vi "ZlutaVanoceVanoce.vi"(11 "NXT/EV3":T1) -> (3 "NXT/EV3 2":T1)   [LabVIEW 2016]
uses:
  <vilib>/NXT/Subs/LVHSConnector.ctl
  <vilib>/NXT/LegoClasses/BrickReference/BrickReference.lvclass
  <vilib>/NXT/Dual Mode Library/Display/drawText_Center.vi
  <vilib>/NXT/Dual Mode Library/Sound/PlayC.vi
  <vilib>/NXT/Dual Mode Library/Sound/PlayA.vi
  <vilib>/NXT/Dual Mode Library/Sound/PlayG.vi
  <vilib>/NXT/Dual Mode Library/Sound/PlayE.vi
  <vilib>/NXT/Dual Mode Library/Sound/PlayD.vi
  <vilib>/NXT/Dual Mode Library/Waits/Wait_Num.vi
  <vilib>/NXT/Dual Mode Library/Sound/PlayB.vi
  <vilib>/NXT/Dual Mode Library/Sound/PlayF.vi
  <vilib>/NXT/Dual Mode Library/Sound/PlayFsharp.vi
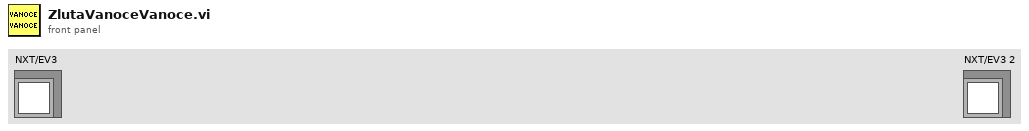
[diagram p1: front panel]
types:
  T1 = typedef "LVHSConnector.ctl" = refnum<class "BrickReference.lvclass">
diagram:
  w7 = u16 5 items=["3"=3, "4"=4, "5"=5, "6"=6, "7"=7] ("Octave")
  w8 = u16 4 items=["3"=3, "4"=4, "5"=5, "6"=6, "7"=7] ("Octave")
  w9 = u16 4 items=["3"=3, "4"=4, "5"=5, "6"=6, "7"=7] ("Octave")
  w10 = u16 4 items=["3"=3, "4"=4, "5"=5, "6"=6, "7"=7] ("Octave")
  w20 = u16 4 items=["3"=3, "4"=4, "5"=5, "6"=6, "7"=7] ("Octave")
  w19 = u16 4 items=["3"=3, "4"=4, "5"=5, "6"=6, "7"=7] ("Octave")
  w47 = u16 4 items=["3"=3, "4"=4, "5"=5, "6"=6, "7"=7] ("Octave")
  w45 = u16 4 items=["3"=3, "4"=4, "5"=5, "6"=6, "7"=7] ("Octave")
  w40 = u16 4 items=["3"=3, "4"=4, "5"=5, "6"=6, "7"=7] ("Octave")
  w39 = u16 4 items=["3"=3, "4"=4, "5"=5, "6"=6, "7"=7] ("Octave")
  w34 = u16 4 items=["3"=3, "4"=4, "5"=5, "6"=6, "7"=7] ("Octave")
  w33 = u16 4 items=["3"=3, "4"=4, "5"=5, "6"=6, "7"=7] ("Octave")
  w32 = u16 4 items=["3"=3, "4"=4, "5"=5, "6"=6, "7"=7] ("Octave")
  w27 = u16 4 items=["3"=3, "4"=4, "5"=5, "6"=6, "7"=7] ("Octave")
  w24 = u16 5 items=["3"=3, "4"=4, "5"=5, "6"=6, "7"=7] ("Octave")
  w23 = u16 5 items=["3"=3, "4"=4, "5"=5, "6"=6, "7"=7] ("Octave")
  w52 = u16 4 items=["3"=3, "4"=4, "5"=5, "6"=6, "7"=7] ("Octave")
  w53 = u16 4 items=["3"=3, "4"=4, "5"=5, "6"=6, "7"=7] ("Octave")
  w54 = u16 4 items=["3"=3, "4"=4, "5"=5, "6"=6, "7"=7] ("Octave")
  w68 = u16 4 items=["3"=3, "4"=4, "5"=5, "6"=6, "7"=7] ("Octave")
  w69 = u16 4 items=["3"=3, "4"=4, "5"=5, "6"=6, "7"=7] ("Octave")
  w70 = u16 4 items=["3"=3, "4"=4, "5"=5, "6"=6, "7"=7] ("Octave")
  w71 = u16 4 items=["3"=3, "4"=4, "5"=5, "6"=6, "7"=7] ("Octave")
  w72 = u16 4 items=["3"=3, "4"=4, "5"=5, "6"=6, "7"=7] ("Octave")
  w73 = u16 4 items=["3"=3, "4"=4, "5"=5, "6"=6, "7"=7] ("Octave")
  w85 = u16 4 items=["3"=3, "4"=4, "5"=5, "6"=6, "7"=7] ("Octave")
  w87 = u16 4 items=["3"=3, "4"=4, "5"=5, "6"=6, "7"=7] ("Octave")
  w92 = u16 4 items=["3"=3, "4"=4, "5"=5, "6"=6, "7"=7] ("Octave")
  w93 = u16 4 items=["3"=3, "4"=4, "5"=5, "6"=6, "7"=7] ("Octave")
  w98 = u16 4 items=["3"=3, "4"=4, "5"=5, "6"=6, "7"=7] ("Octave")
  w99 = u16 4 items=["3"=3, "4"=4, "5"=5, "6"=6, "7"=7] ("Octave")
  w100 = u16 4 items=["3"=3, "4"=4, "5"=5, "6"=6, "7"=7] ("Octave")
  w106 = u16 4 items=["3"=3, "4"=4, "5"=5, "6"=6, "7"=7] ("Octave")
  w109 = u16 5 items=["3"=3, "4"=4, "5"=5, "6"=6, "7"=7] ("Octave")
  w110 = u16 5 items=["3"=3, "4"=4, "5"=5, "6"=6, "7"=7] ("Octave")
  w115 = u16 4 items=["3"=3, "4"=4, "5"=5, "6"=6, "7"=7] ("Octave")
  w118 = u16 4 items=["3"=3, "4"=4, "5"=5, "6"=6, "7"=7] ("Octave")
  w119 = u16 4 items=["3"=3, "4"=4, "5"=5, "6"=6, "7"=7] ("Octave")
  w145 = u16 4 items=["3"=3, "4"=4, "5"=5, "6"=6, "7"=7] ("Octave")
  w149 = u16 4 items=["3"=3, "4"=4, "5"=5, "6"=6, "7"=7] ("Octave")
  w146 = u16 4 items=["3"=3, "4"=4, "5"=5, "6"=6, "7"=7] ("Octave")
  w138 = u16 4 items=["3"=3, "4"=4, "5"=5, "6"=6, "7"=7] ("Octave")
  w135 = u16 4 items=["3"=3, "4"=4, "5"=5, "6"=6, "7"=7] ("Octave")
  w130 = u16 4 items=["3"=3, "4"=4, "5"=5, "6"=6, "7"=7] ("Octave")
  w133 = u16 4 items=["3"=3, "4"=4, "5"=5, "6"=6, "7"=7] ("Octave")
  w125 = u16 4 items=["3"=3, "4"=4, "5"=5, "6"=6, "7"=7] ("Octave")
  w122 = u16 4 items=["3"=3, "4"=4, "5"=5, "6"=6, "7"=7] ("Octave")
  w121 = u16 4 items=["3"=3, "4"=4, "5"=5, "6"=6, "7"=7] ("Octave")
  w167 = u16 4 items=["3"=3, "4"=4, "5"=5, "6"=6, "7"=7] ("Octave")
  w164 = u16 4 items=["3"=3, "4"=4, "5"=5, "6"=6, "7"=7] ("Octave")
  w160 = u16 4 items=["3"=3, "4"=4, "5"=5, "6"=6, "7"=7] ("Octave")
  w163 = u16 4 items=["3"=3, "4"=4, "5"=5, "6"=6, "7"=7] ("Octave")
  w175 = u16 4 items=["3"=3, "4"=4, "5"=5, "6"=6, "7"=7] ("Octave")
  w178 = u16 4 items=["3"=3, "4"=4, "5"=5, "6"=6, "7"=7] ("Octave")
  w183 = u16 4 items=["3"=3, "4"=4, "5"=5, "6"=6, "7"=7] ("Octave")
  w180 = u16 4 items=["3"=3, "4"=4, "5"=5, "6"=6, "7"=7] ("Octave")
  w188 = u16 4 items=["3"=3, "4"=4, "5"=5, "6"=6, "7"=7] ("Octave")
  w191 = u16 4 items=["3"=3, "4"=4, "5"=5, "6"=6, "7"=7] ("Octave")
  w192 = u16 4 items=["3"=3, "4"=4, "5"=5, "6"=6, "7"=7] ("Octave")
  w195 = u16 4 items=["3"=3, "4"=4, "5"=5, "6"=6, "7"=7] ("Octave")
  w203 = u16 5 items=["3"=3, "4"=4, "5"=5, "6"=6, "7"=7] ("Octave")
  w204 = u16 4 items=["3"=3, "4"=4, "5"=5, "6"=6, "7"=7] ("Octave")
  w205 = u16 4 items=["3"=3, "4"=4, "5"=5, "6"=6, "7"=7] ("Octave")
  w206 = u16 4 items=["3"=3, "4"=4, "5"=5, "6"=6, "7"=7] ("Octave")
  w216 = u16 4 items=["3"=3, "4"=4, "5"=5, "6"=6, "7"=7] ("Octave")
  w215 = u16 4 items=["3"=3, "4"=4, "5"=5, "6"=6, "7"=7] ("Octave")
  w243 = u16 4 items=["3"=3, "4"=4, "5"=5, "6"=6, "7"=7] ("Octave")
  w241 = u16 4 items=["3"=3, "4"=4, "5"=5, "6"=6, "7"=7] ("Octave")
  w236 = u16 4 items=["3"=3, "4"=4, "5"=5, "6"=6, "7"=7] ("Octave")
  w235 = u16 4 items=["3"=3, "4"=4, "5"=5, "6"=6, "7"=7] ("Octave")
  w230 = u16 4 items=["3"=3, "4"=4, "5"=5, "6"=6, "7"=7] ("Octave")
  w229 = u16 4 items=["3"=3, "4"=4, "5"=5, "6"=6, "7"=7] ("Octave")
  w228 = u16 4 items=["3"=3, "4"=4, "5"=5, "6"=6, "7"=7] ("Octave")
  w223 = u16 4 items=["3"=3, "4"=4, "5"=5, "6"=6, "7"=7] ("Octave")
  w220 = u16 5 items=["3"=3, "4"=4, "5"=5, "6"=6, "7"=7] ("Octave")
  w219 = u16 5 items=["3"=3, "4"=4, "5"=5, "6"=6, "7"=7] ("Octave")
  w248 = u16 4 items=["3"=3, "4"=4, "5"=5, "6"=6, "7"=7] ("Octave")
  w249 = u16 4 items=["3"=3, "4"=4, "5"=5, "6"=6, "7"=7] ("Octave")
  w250 = u16 4 items=["3"=3, "4"=4, "5"=5, "6"=6, "7"=7] ("Octave")
  w264 = u16 4 items=["3"=3, "4"=4, "5"=5, "6"=6, "7"=7] ("Octave")
  w265 = u16 4 items=["3"=3, "4"=4, "5"=5, "6"=6, "7"=7] ("Octave")
  w266 = u16 4 items=["3"=3, "4"=4, "5"=5, "6"=6, "7"=7] ("Octave")
  w267 = u16 4 items=["3"=3, "4"=4, "5"=5, "6"=6, "7"=7] ("Octave")
  w268 = u16 4 items=["3"=3, "4"=4, "5"=5, "6"=6, "7"=7] ("Octave")
  w269 = u16 4 items=["3"=3, "4"=4, "5"=5, "6"=6, "7"=7] ("Octave")
  w279 = i16 0 items=["1", "2", "3", "4", "5", "6", "7", "8", "9", "10", "11", "12"] ("Line")
  w283 = u16 4 items=["3"=3, "4"=4, "5"=5, "6"=6, "7"=7] ("Octave")
  w285 = u16 4 items=["3"=3, "4"=4, "5"=5, "6"=6, "7"=7] ("Octave")
  w290 = u16 4 items=["3"=3, "4"=4, "5"=5, "6"=6, "7"=7] ("Octave")
  w291 = u16 4 items=["3"=3, "4"=4, "5"=5, "6"=6, "7"=7] ("Octave")
  w296 = u16 4 items=["3"=3, "4"=4, "5"=5, "6"=6, "7"=7] ("Octave")
  w297 = u16 4 items=["3"=3, "4"=4, "5"=5, "6"=6, "7"=7] ("Octave")
  w298 = u16 4 items=["3"=3, "4"=4, "5"=5, "6"=6, "7"=7] ("Octave")
  w304 = u16 4 items=["3"=3, "4"=4, "5"=5, "6"=6, "7"=7] ("Octave")
  w307 = u16 5 items=["3"=3, "4"=4, "5"=5, "6"=6, "7"=7] ("Octave")
  w308 = u16 5 items=["3"=3, "4"=4, "5"=5, "6"=6, "7"=7] ("Octave")
  n1 = call-poly <vilib>:"PolyDisplay.vi"("Text"="\n\n\n\n\nEV3 JUK3BOX:\nVanoce, Vanoce\n\n\n\n\n\n", "NXT/EV3"="NXT/EV3", "Line"=w279) -> ("NXT/EV3"=w196:T1)  [unwired: 1 in]
  n2 = call-poly <vilib>:"PolySound.vi"("Duration (500 ms)"=u16 1000, "NXT/EV3"=w196, "Octave"=w308) -> ("NXT/EV3"=w303:T1)  [unwired: 1 in]
  n3 = call-poly <vilib>:"PolySound.vi"("Duration (500 ms)"=u16 500, "NXT/EV3"=w303, "Octave"=w307) -> ("NXT/EV3"=w302:T1)  [unwired: 1 in]
  n4 = call-poly <vilib>:"PolySound.vi"("Duration (500 ms)"=u16 500, "NXT/EV3"=w302, "Octave"=w304) -> ("NXT/EV3"=w301:T1)  [unwired: 1 in]
  n5 = call-poly <vilib>:"PolySound.vi"("Duration (500 ms)"=u16 1000, "NXT/EV3"=w301, "Octave"=w298) -> ("NXT/EV3"=w300:T1)  [unwired: 1 in]
  n6 = call-poly <vilib>:"PolySound.vi"("Duration (500 ms)"=u16 500, "NXT/EV3"=w300, "Octave"=w297) -> ("NXT/EV3"=w299:T1)  [unwired: 1 in]
  n7 = call-poly <vilib>:"PolySound.vi"("Duration (500 ms)"=u16 500, "NXT/EV3"=w299, "Octave"=w296) -> ("NXT/EV3"=w288:T1)  [unwired: 1 in]
  n8 = call-poly <vilib>:"PolySound.vi"("Duration (500 ms)"=u16 500, "NXT/EV3"=w288, "Octave"=w291) -> ("NXT/EV3"=w287:T1)  [unwired: 1 in]
  n9 = call-poly <vilib>:"PolySound.vi"("Duration (500 ms)"=u16 1000, "NXT/EV3"=w287, "Octave"=w290) -> ("NXT/EV3"=w284:T1)  [unwired: 1 in]
  n10 = call-poly <vilib>:"PolySound.vi"("Duration (500 ms)"=u16 500, "NXT/EV3"=w284, "Octave"=w285) -> ("NXT/EV3"=w282:T1)  [unwired: 1 in]
  n11 = call-poly <vilib>:"PolySound.vi"("Duration (500 ms)"=u16 1000, "NXT/EV3"=w282, "Octave"=w283) -> ("NXT/EV3"=w261:T1)  [unwired: 1 in]
  n12 = call-poly <vilib>:"PolyWait.vi"("Time (1 sec)"=sgl 0.7, "NXT/EV3"=w261) -> ("NXT/EV3"=w260:T1)  [unwired: 2 in]
  n13 = call-poly <vilib>:"PolySound.vi"("Duration (500 ms)"=u16 500, "NXT/EV3"=w260, "Octave"=w269) -> ("NXT/EV3"=w278:T1)  [unwired: 1 in]
  n14 = call-poly <vilib>:"PolySound.vi"("Duration (500 ms)"=u16 1000, "NXT/EV3"=w278, "Octave"=w268) -> ("NXT/EV3"=w277:T1)  [unwired: 1 in]
  n15 = call-poly <vilib>:"PolySound.vi"("Duration (500 ms)"=u16 500, "NXT/EV3"=w277, "Octave"=w267) -> ("NXT/EV3"=w276:T1)  [unwired: 1 in]
  n16 = call-poly <vilib>:"PolySound.vi"("Duration (500 ms)"=u16 1000, "NXT/EV3"=w276, "Octave"=w266) -> ("NXT/EV3"=w275:T1)  [unwired: 1 in]
  n17 = call-poly <vilib>:"PolySound.vi"("Duration (500 ms)"=u16 1000, "NXT/EV3"=w275, "Octave"=w265) -> ("NXT/EV3"=w262:T1)  [unwired: 1 in]
  n18 = call-poly <vilib>:"PolySound.vi"("Duration (500 ms)"=u16 1900, "NXT/EV3"=w262, "Octave"=w264) -> ("NXT/EV3"=w258:T1)  [unwired: 1 in]
  n19 = call-poly <vilib>:"PolyWait.vi"("Time (1 sec)"=sgl 0.3, "NXT/EV3"=w258) -> ("NXT/EV3"=w256:T1)  [unwired: 2 in]
  n20 = call-poly <vilib>:"PolySound.vi"("Duration (500 ms)"=u16 500, "NXT/EV3"=w256, "Octave"=w250) -> ("NXT/EV3"=w255:T1)  [unwired: 1 in]
  n21 = call-poly <vilib>:"PolySound.vi"("Duration (500 ms)"=u16 500, "NXT/EV3"=w255, "Octave"=w249) -> ("NXT/EV3"=w254:T1)  [unwired: 1 in]
  n22 = call-poly <vilib>:"PolySound.vi"("Duration (500 ms)"=u16 500, "NXT/EV3"=w254, "Octave"=w248) -> ("NXT/EV3"=w217:T1)  [unwired: 1 in]
  n23 = call-poly <vilib>:"PolySound.vi"("Duration (500 ms)"=u16 1000, "NXT/EV3"=w217, "Octave"=w219) -> ("NXT/EV3"=w224:T1)  [unwired: 1 in]
  n24 = call-poly <vilib>:"PolySound.vi"("Duration (500 ms)"=u16 500, "NXT/EV3"=w224, "Octave"=w220) -> ("NXT/EV3"=w197:T1)  [unwired: 1 in]
  "NXT/EV3 2" <- w197
  n25 = call-poly <vilib>:"PolySound.vi"("Duration (500 ms)"=u16 500, "NXT/EV3"=w197, "Octave"=w223) -> ("NXT/EV3"=w225:T1)  [unwired: 1 in]
  n26 = call-poly <vilib>:"PolySound.vi"("Duration (500 ms)"=u16 1000, "NXT/EV3"=w225, "Octave"=w228) -> ("NXT/EV3"=w226:T1)  [unwired: 1 in]
  n27 = call-poly <vilib>:"PolySound.vi"("Duration (500 ms)"=u16 500, "NXT/EV3"=w226, "Octave"=w229) -> ("NXT/EV3"=w227:T1)  [unwired: 1 in]
  n28 = call-poly <vilib>:"PolySound.vi"("Duration (500 ms)"=u16 500, "NXT/EV3"=w227, "Octave"=w230) -> ("NXT/EV3"=w238:T1)  [unwired: 1 in]
  n29 = call-poly <vilib>:"PolySound.vi"("Duration (500 ms)"=u16 500, "NXT/EV3"=w238, "Octave"=w235) -> ("NXT/EV3"=w239:T1)  [unwired: 1 in]
  n30 = call-poly <vilib>:"PolySound.vi"("Duration (500 ms)"=u16 1000, "NXT/EV3"=w239, "Octave"=w236) -> ("NXT/EV3"=w242:T1)  [unwired: 1 in]
  n31 = call-poly <vilib>:"PolySound.vi"("Duration (500 ms)"=u16 500, "NXT/EV3"=w242, "Octave"=w241) -> ("NXT/EV3"=w244:T1)  [unwired: 1 in]
  n32 = call-poly <vilib>:"PolySound.vi"("Duration (500 ms)"=u16 1000, "NXT/EV3"=w244, "Octave"=w243) -> ("NXT/EV3"=w246:T1)  [unwired: 1 in]
  n33 = call-poly <vilib>:"PolyWait.vi"("Time (1 sec)"=sgl 0.7, "NXT/EV3"=w246) -> ("NXT/EV3"=w211:T1)  [unwired: 2 in]
  n34 = call-poly <vilib>:"PolySound.vi"("Duration (500 ms)"=u16 500, "NXT/EV3"=w211, "Octave"=w215) -> ("NXT/EV3"=w212:T1)  [unwired: 1 in]
  n35 = call-poly <vilib>:"PolySound.vi"("Duration (500 ms)"=u16 1000, "NXT/EV3"=w212, "Octave"=w216) -> ("NXT/EV3"=w210:T1)  [unwired: 1 in]
  n36 = call-poly <vilib>:"PolySound.vi"("Duration (500 ms)"=u16 500, "NXT/EV3"=w210, "Octave"=w206) -> ("NXT/EV3"=w209:T1)  [unwired: 1 in]
  n37 = call-poly <vilib>:"PolySound.vi"("Duration (500 ms)"=u16 1000, "NXT/EV3"=w209, "Octave"=w205) -> ("NXT/EV3"=w208:T1)  [unwired: 1 in]
  n38 = call-poly <vilib>:"PolySound.vi"("Duration (500 ms)"=u16 1000, "NXT/EV3"=w208, "Octave"=w204) -> ("NXT/EV3"=w207:T1)  [unwired: 1 in]
  n39 = call-poly <vilib>:"PolySound.vi"("Duration (500 ms)"=u16 2000, "NXT/EV3"=w207, "Octave"=w203) -> ("NXT/EV3"=w172:T1)  [unwired: 1 in]
  n40 = call-poly <vilib>:"PolyWait.vi"("Time (1 sec)"=sgl 0.7, "NXT/EV3"=w172) -> ("NXT/EV3"=w171:T1)  [unwired: 2 in]
  n41 = call-poly <vilib>:"PolySound.vi"("Duration (500 ms)"=u16 500, "NXT/EV3"=w171, "Octave"=w195) -> ("NXT/EV3"=w187:T1)  [unwired: 1 in]
  n42 = call-poly <vilib>:"PolySound.vi"("Duration (500 ms)"=u16 500, "NXT/EV3"=w187, "Octave"=w192) -> ("NXT/EV3"=w186:T1)  [unwired: 1 in]
  n43 = call-poly <vilib>:"PolySound.vi"("Duration (500 ms)"=u16 500, "NXT/EV3"=w186, "Octave"=w191) -> ("NXT/EV3"=w185:T1)  [unwired: 1 in]
  n44 = call-poly <vilib>:"PolySound.vi"("Duration (500 ms)"=u16 500, "NXT/EV3"=w185, "Octave"=w188) -> ("NXT/EV3"=w179:T1)  [unwired: 1 in]
  n45 = call-poly <vilib>:"PolySound.vi"("Duration (500 ms)"=u16 500, "NXT/EV3"=w179, "Octave"=w180) -> ("NXT/EV3"=w184:T1)  [unwired: 1 in]
  n46 = call-poly <vilib>:"PolySound.vi"("Duration (500 ms)"=u16 500, "NXT/EV3"=w184, "Octave"=w183) -> ("NXT/EV3"=w173:T1)  [unwired: 1 in]
  n47 = call-poly <vilib>:"PolySound.vi"("Duration (500 ms)"=u16 500, "NXT/EV3"=w173, "Octave"=w178) -> ("NXT/EV3"=w174:T1)  [unwired: 1 in]
  n48 = call-poly <vilib>:"PolySound.vi"("Duration (500 ms)"=u16 500, "NXT/EV3"=w174, "Octave"=w175) -> ("NXT/EV3"=w158:T1)  [unwired: 1 in]
  n49 = call-poly <vilib>:"PolySound.vi"("Duration (500 ms)"=u16 500, "NXT/EV3"=w158, "Octave"=w163) -> ("NXT/EV3"=w159:T1)  [unwired: 1 in]
  n50 = call-poly <vilib>:"PolySound.vi"("Duration (500 ms)"=u16 500, "NXT/EV3"=w159, "Octave"=w160) -> ("NXT/EV3"=w169:T1)  [unwired: 1 in]
  n51 = call-poly <vilib>:"PolySound.vi"("Duration (500 ms)"=u16 500, "NXT/EV3"=w169, "Octave"=w164) -> ("NXT/EV3"=w168:T1)  [unwired: 1 in]
  n52 = call-poly <vilib>:"PolySound.vi"("Duration (500 ms)"=u16 500, "NXT/EV3"=w168, "Octave"=w167) -> ("NXT/EV3"=w157:T1)  [unwired: 1 in]
  n53 = call-poly <vilib>:"PolySound.vi"("Duration (500 ms)"=u16 500, "NXT/EV3"=w157) -> ("NXT/EV3"=w156:T1)  [unwired: 2 in]
  n54 = call-poly <vilib>:"PolySound.vi"("Duration (500 ms)"=u16 500, "NXT/EV3"=w156) -> ("NXT/EV3"=w155:T1)  [unwired: 2 in]
  n55 = call-poly <vilib>:"PolySound.vi"("Duration (500 ms)"=u16 750, "NXT/EV3"=w155) -> ("NXT/EV3"=w117:T1)  [unwired: 2 in]
  n56 = call-poly <vilib>:"PolySound.vi"("NXT/EV3"=w117, "Octave"=w118) -> ("NXT/EV3"=w126:T1)  [unwired: 2 in]
  n57 = call-poly <vilib>:"PolySound.vi"("Duration (500 ms)"=u16 500, "NXT/EV3"=w126, "Octave"=w121) -> ("NXT/EV3"=w127:T1)  [unwired: 1 in]
  n58 = call-poly <vilib>:"PolySound.vi"("Duration (500 ms)"=u16 500, "NXT/EV3"=w127, "Octave"=w122) -> ("NXT/EV3"=w128:T1)  [unwired: 1 in]
  n59 = call-poly <vilib>:"PolySound.vi"("Duration (500 ms)"=u16 500, "NXT/EV3"=w128, "Octave"=w125) -> ("NXT/EV3"=w134:T1)  [unwired: 1 in]
  n60 = call-poly <vilib>:"PolySound.vi"("Duration (500 ms)"=u16 500, "NXT/EV3"=w134, "Octave"=w133) -> ("NXT/EV3"=w129:T1)  [unwired: 1 in]
  n61 = call-poly <vilib>:"PolySound.vi"("Duration (500 ms)"=u16 500, "NXT/EV3"=w129, "Octave"=w130) -> ("NXT/EV3"=w140:T1)  [unwired: 1 in]
  n62 = call-poly <vilib>:"PolySound.vi"("Duration (500 ms)"=u16 500, "NXT/EV3"=w140, "Octave"=w135) -> ("NXT/EV3"=w139:T1)  [unwired: 1 in]
  n63 = call-poly <vilib>:"PolySound.vi"("Duration (500 ms)"=u16 500, "NXT/EV3"=w139, "Octave"=w138) -> ("NXT/EV3"=w151:T1)  [unwired: 1 in]
  n64 = call-poly <vilib>:"PolySound.vi"("Duration (500 ms)"=u16 500, "NXT/EV3"=w151, "Octave"=w146) -> ("NXT/EV3"=w150:T1)  [unwired: 1 in]
  n65 = call-poly <vilib>:"PolySound.vi"("Duration (500 ms)"=u16 500, "NXT/EV3"=w150, "Octave"=w149) -> ("NXT/EV3"=w141:T1)  [unwired: 1 in]
  n66 = call-poly <vilib>:"PolySound.vi"("Duration (500 ms)"=u16 500, "NXT/EV3"=w141, "Octave"=w145) -> ("NXT/EV3"=w142:T1)  [unwired: 1 in]
  n67 = call-poly <vilib>:"PolySound.vi"("Duration (500 ms)"=u16 500, "NXT/EV3"=w142, "Octave"=w119) -> ("NXT/EV3"=w114:T1)  [unwired: 1 in]
  n68 = call-poly <vilib>:"PolySound.vi"("Duration (500 ms)"=u16 750, "NXT/EV3"=w114, "Octave"=w115) -> ("NXT/EV3"=w113:T1)  [unwired: 1 in]
  n69 = call-poly <vilib>:"PolyWait.vi"("Time (1 sec)"=sgl 0.75, "NXT/EV3"=w113) -> ("NXT/EV3"=w1:T1)  [unwired: 2 in]
  n70 = call-poly <vilib>:"PolySound.vi"("Duration (500 ms)"=u16 1000, "NXT/EV3"=w1, "Octave"=w110) -> ("NXT/EV3"=w105:T1)  [unwired: 1 in]
  n71 = call-poly <vilib>:"PolySound.vi"("Duration (500 ms)"=u16 500, "NXT/EV3"=w105, "Octave"=w109) -> ("NXT/EV3"=w104:T1)  [unwired: 1 in]
  n72 = call-poly <vilib>:"PolySound.vi"("Duration (500 ms)"=u16 500, "NXT/EV3"=w104, "Octave"=w106) -> ("NXT/EV3"=w103:T1)  [unwired: 1 in]
  n73 = call-poly <vilib>:"PolySound.vi"("Duration (500 ms)"=u16 1000, "NXT/EV3"=w103, "Octave"=w100) -> ("NXT/EV3"=w102:T1)  [unwired: 1 in]
  n74 = call-poly <vilib>:"PolySound.vi"("Duration (500 ms)"=u16 500, "NXT/EV3"=w102, "Octave"=w99) -> ("NXT/EV3"=w101:T1)  [unwired: 1 in]
  n75 = call-poly <vilib>:"PolySound.vi"("Duration (500 ms)"=u16 500, "NXT/EV3"=w101, "Octave"=w98) -> ("NXT/EV3"=w90:T1)  [unwired: 1 in]
  n76 = call-poly <vilib>:"PolySound.vi"("Duration (500 ms)"=u16 500, "NXT/EV3"=w90, "Octave"=w93) -> ("NXT/EV3"=w89:T1)  [unwired: 1 in]
  n77 = call-poly <vilib>:"PolySound.vi"("Duration (500 ms)"=u16 1000, "NXT/EV3"=w89, "Octave"=w92) -> ("NXT/EV3"=w86:T1)  [unwired: 1 in]
  n78 = call-poly <vilib>:"PolySound.vi"("Duration (500 ms)"=u16 500, "NXT/EV3"=w86, "Octave"=w87) -> ("NXT/EV3"=w84:T1)  [unwired: 1 in]
  n79 = call-poly <vilib>:"PolySound.vi"("Duration (500 ms)"=u16 1000, "NXT/EV3"=w84, "Octave"=w85) -> ("NXT/EV3"=w65:T1)  [unwired: 1 in]
  n80 = call-poly <vilib>:"PolyWait.vi"("Time (1 sec)"=sgl 0.7, "NXT/EV3"=w65) -> ("NXT/EV3"=w64:T1)  [unwired: 2 in]
  n81 = call-poly <vilib>:"PolySound.vi"("Duration (500 ms)"=u16 500, "NXT/EV3"=w64, "Octave"=w73) -> ("NXT/EV3"=w82:T1)  [unwired: 1 in]
  n82 = call-poly <vilib>:"PolySound.vi"("Duration (500 ms)"=u16 1000, "NXT/EV3"=w82, "Octave"=w72) -> ("NXT/EV3"=w81:T1)  [unwired: 1 in]
  n83 = call-poly <vilib>:"PolySound.vi"("Duration (500 ms)"=u16 500, "NXT/EV3"=w81, "Octave"=w71) -> ("NXT/EV3"=w80:T1)  [unwired: 1 in]
  n84 = call-poly <vilib>:"PolySound.vi"("Duration (500 ms)"=u16 1000, "NXT/EV3"=w80, "Octave"=w70) -> ("NXT/EV3"=w79:T1)  [unwired: 1 in]
  n85 = call-poly <vilib>:"PolySound.vi"("Duration (500 ms)"=u16 1000, "NXT/EV3"=w79, "Octave"=w69) -> ("NXT/EV3"=w66:T1)  [unwired: 1 in]
  n86 = call-poly <vilib>:"PolySound.vi"("Duration (500 ms)"=u16 1900, "NXT/EV3"=w66, "Octave"=w68) -> ("NXT/EV3"=w62:T1)  [unwired: 1 in]
  n87 = call-poly <vilib>:"PolyWait.vi"("Time (1 sec)"=sgl 0.3, "NXT/EV3"=w62) -> ("NXT/EV3"=w60:T1)  [unwired: 2 in]
  n88 = call-poly <vilib>:"PolySound.vi"("Duration (500 ms)"=u16 500, "NXT/EV3"=w60, "Octave"=w54) -> ("NXT/EV3"=w59:T1)  [unwired: 1 in]
  n89 = call-poly <vilib>:"PolySound.vi"("Duration (500 ms)"=u16 500, "NXT/EV3"=w59, "Octave"=w53) -> ("NXT/EV3"=w58:T1)  [unwired: 1 in]
  n90 = call-poly <vilib>:"PolySound.vi"("Duration (500 ms)"=u16 500, "NXT/EV3"=w58, "Octave"=w52) -> ("NXT/EV3"=w21:T1)  [unwired: 1 in]
  n91 = call-poly <vilib>:"PolySound.vi"("Duration (500 ms)"=u16 1000, "NXT/EV3"=w21, "Octave"=w23) -> ("NXT/EV3"=w28:T1)  [unwired: 1 in]
  n92 = call-poly <vilib>:"PolySound.vi"("Duration (500 ms)"=u16 500, "NXT/EV3"=w28, "Octave"=w24) -> ("NXT/EV3"=w2:T1)  [unwired: 1 in]
  n93 = call-poly <vilib>:"PolySound.vi"("Duration (500 ms)"=u16 500, "NXT/EV3"=w2, "Octave"=w27) -> ("NXT/EV3"=w29:T1)  [unwired: 1 in]
  n94 = call-poly <vilib>:"PolySound.vi"("Duration (500 ms)"=u16 1000, "NXT/EV3"=w29, "Octave"=w32) -> ("NXT/EV3"=w30:T1)  [unwired: 1 in]
  n95 = call-poly <vilib>:"PolySound.vi"("Duration (500 ms)"=u16 500, "NXT/EV3"=w30, "Octave"=w33) -> ("NXT/EV3"=w31:T1)  [unwired: 1 in]
  n96 = call-poly <vilib>:"PolySound.vi"("Duration (500 ms)"=u16 500, "NXT/EV3"=w31, "Octave"=w34) -> ("NXT/EV3"=w42:T1)  [unwired: 1 in]
  n97 = call-poly <vilib>:"PolySound.vi"("Duration (500 ms)"=u16 500, "NXT/EV3"=w42, "Octave"=w39) -> ("NXT/EV3"=w43:T1)  [unwired: 1 in]
  n98 = call-poly <vilib>:"PolySound.vi"("Duration (500 ms)"=u16 1000, "NXT/EV3"=w43, "Octave"=w40) -> ("NXT/EV3"=w46:T1)  [unwired: 1 in]
  n99 = call-poly <vilib>:"PolySound.vi"("Duration (500 ms)"=u16 500, "NXT/EV3"=w46, "Octave"=w45) -> ("NXT/EV3"=w48:T1)  [unwired: 1 in]
  n100 = call-poly <vilib>:"PolySound.vi"("Duration (500 ms)"=u16 1000, "NXT/EV3"=w48, "Octave"=w47) -> ("NXT/EV3"=w50:T1)  [unwired: 1 in]
  n101 = call-poly <vilib>:"PolyWait.vi"("Time (1 sec)"=sgl 0.7, "NXT/EV3"=w50) -> ("NXT/EV3"=w15:T1)  [unwired: 2 in]
  n102 = call-poly <vilib>:"PolySound.vi"("Duration (500 ms)"=u16 500, "NXT/EV3"=w15, "Octave"=w19) -> ("NXT/EV3"=w16:T1)  [unwired: 1 in]
  n103 = call-poly <vilib>:"PolySound.vi"("Duration (500 ms)"=u16 1000, "NXT/EV3"=w16, "Octave"=w20) -> ("NXT/EV3"=w14:T1)  [unwired: 1 in]
  n104 = call-poly <vilib>:"PolySound.vi"("Duration (500 ms)"=u16 500, "NXT/EV3"=w14, "Octave"=w10) -> ("NXT/EV3"=w13:T1)  [unwired: 1 in]
  n105 = call-poly <vilib>:"PolySound.vi"("Duration (500 ms)"=u16 1000, "NXT/EV3"=w13, "Octave"=w9) -> ("NXT/EV3"=w12:T1)  [unwired: 1 in]
  n106 = call-poly <vilib>:"PolySound.vi"("Duration (500 ms)"=u16 1000, "NXT/EV3"=w12, "Octave"=w8) -> ("NXT/EV3"=w11:T1)  [unwired: 1 in]
  n107 = call-poly <vilib>:"PolySound.vi"("Duration (500 ms)"=u16 2000, "NXT/EV3"=w11, "Octave"=w7) -> ()  [unwired: 1 in, 1 out]
